vi "CRYGet DataView ToolBar Ref.vi"(11 "DataViewb in":T1) -> (3 "pRefListTF_Out":refnum<vi>[](array[refnum]))   [LabVIEW 2013]
uses:
  Control/Graph Main Info Cluster.ctl
  Control/SplitterBar.ctl
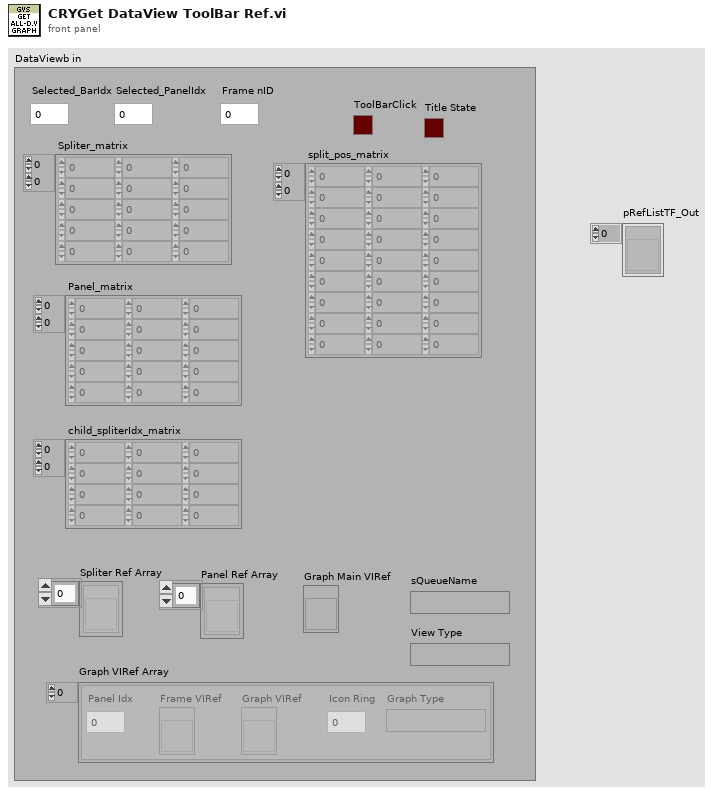
[diagram p1: front panel]
types:
  T1 = typedef "Graph Main Info Cluster.ctl" = cluster{"Selected_BarIdx":i32, "Selected_PanelIdx":i32, "Graph Main VIRef":refnum<vi>, "ToolBarClick":bool, "Spliter Ref Array":refnum<vi>[], "Panel Ref Array":refnum<vi>[], "Spliter_matrix":i32[][], "Panel_matrix":i32[][], "child_spliterIdx_matrix":i32[][], "split_pos_matrix":i32[][], "Title State":bool, "sQueueName":string, "Frame nID":i32, "Graph VIRef Array":cluster{"Graph VIRef":refnum<vi>, "Panel Idx":i32, "Frame VIRef":refnum<vi>, "Icon Ring":i32, "Graph Type":string}[], "View Type":string}
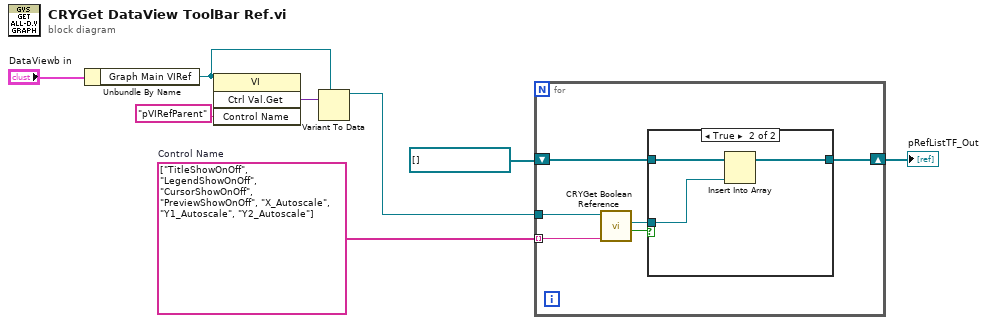
[diagram p0: block diagram]
diagram:
  w7 = string[] ["TitleShowOnOff", "LegendShowOnOff", "CursorShowOnOff", "PreviewShowOnOff", "X_Autoscale", "Y1_Autoscale", "Y2_Autoscale"]  # Control Name
  n1 = Unbundle By Name("DataViewb in") -> ("Graph Main VIRef"=w2:refnum<vi>)
  n2 = invoke class="VI" method="Ctrl Val.Get"(reference=w2, "Control Name"="pVIRefParent") -> ("Get Control Value Variant"=w3:variant)  [unwired: 2 in, 3 out]
  n3 = Variant To Data(type=w2, Variant=w3) -> (data=w1:refnum<vi>)  [unwired: 1 in, 1 out]
  n4 = for {
    tunnel: w7 -> [w13] mode=indexing
    tunnel: w1 -> [w14]
    shift-right: [w9] -> w5
    shift-left: refnum<vi>[] [] ("pRefListTF_Out") -> [w10]
    n5 = call "CRYGet Boolean Reference.vi"("Label Name"=w13, "VI Refnum"=w14) -> ("Exist?"=w12:bool, "Boolean Ref"=w11:refnum<vi>)  [unwired: 7 in, 1 out]
    n6 = case shown="True" w12 {
      tunnel: w11 -> [_ w17]
      tunnel: w10 -> [w15 w18]
      tunnel: [w15 w16] -> w9
      frame False {
      }
      frame True {
        n7 = Insert Into Array(array=w18, new element=w17) -> (w16:refnum<vi>[])  [unwired: 1 in]
      }
    }
  }
  "pRefListTF_Out" <- w5
